vi "Start.vi"(8 "error in (no error)":errorcluster, 11 "Transceiver Thread in":refnum<class "Transceiver Thread.lvclass">) -> (0 "error out":errorcluster, 3 "Transceiver Thread out":refnum<class "Transceiver Thread.lvclass">)   [LabVIEW 2017, in "DSF Core.lvlib" / "Transceiver Thread.lvclass"]
uses:
  Transceiver Thread.lvclass
  Transceiver Thread.lvclass/Transceiver Thread.ctl
  Transceiver/Transceiver.lvclass
  Buffer Converter/Buffer Converter.lvclass
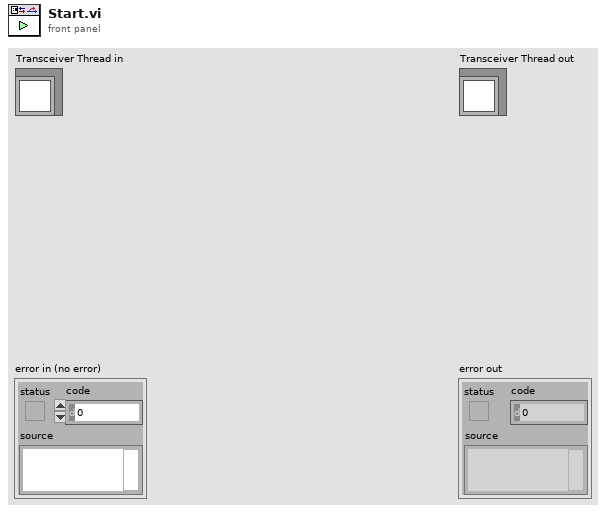
[diagram p1: front panel]
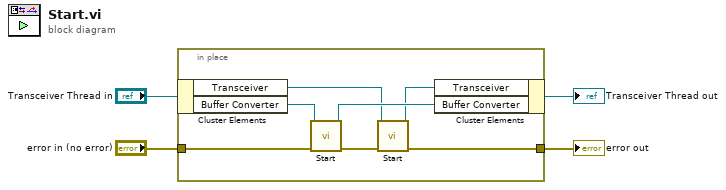
[diagram p0: block diagram]
diagram:
  n1 = in-place {
    in-place-border: "error in (no error)" -> [w10]
    in-place-border: [w5] -> w2
    n2 = in-place-cluster #1("Transceiver Thread in") -> ("Transceiver"=w7:refnum<class "Transceiver.lvclass">, "Buffer Converter"=w11:refnum<class "Buffer Converter.lvclass">)
    n3 = call-dynamic "Start.vi"("error in (no error)"=w10, "Buffer Converter in"=w11) -> ("error out"=w9:errorcluster, "Buffer Converter out"=w8:refnum<class "Buffer Converter.lvclass">)  [unwired: 8 in]
    n4 = call-dynamic "Start.vi"("error in (no error)"=w9, "Transceiver in"=w7) -> ("error out"=w5:errorcluster, "Transceiver out"=w6:refnum<class "Transceiver.lvclass">)  [unwired: 8 in]
    n5 = in-place-cluster #1("Transceiver"=w6, "Buffer Converter"=w8) -> (→"Transceiver Thread out":refnum<class "Transceiver Thread.lvclass">)
  }
  "error out" <- w2
